vi "setSettingControlReferences.vi"(10 "SettingControlReferences":refnum<vi>[](array[refnum]), 11 "Setting in":refnum<class "Setting.lvclass">) -> (3 "Setting out":refnum<class "Setting.lvclass">)   [LabVIEW 2020, in "Settings.lvlib" / "Setting.lvclass"]
uses:
  Setting.lvclass
  Setting.lvclass/Setting.ctl
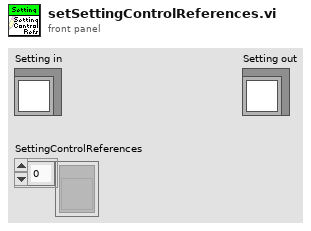
[diagram p1: front panel]
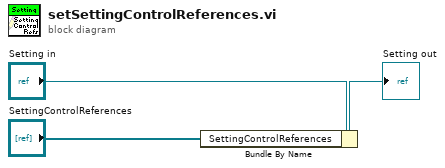
[diagram p0: block diagram]
diagram:
  n1 = Bundle By Name(cluster="Setting in", "SettingControlReferences"="SettingControlReferences") -> (→"Setting out":refnum<class "Setting.lvclass">)
